vi "IO_csv_writer.vi"(0 "info_sheet":string, 1 "path":path, 2 "y_data_arr":dbl[][](array[numeric]), 3 "x_data_arr":dbl[][](array[numeric])) -> ()   [LabVIEW 2014]
uses:
  dll/csv_operator.dll
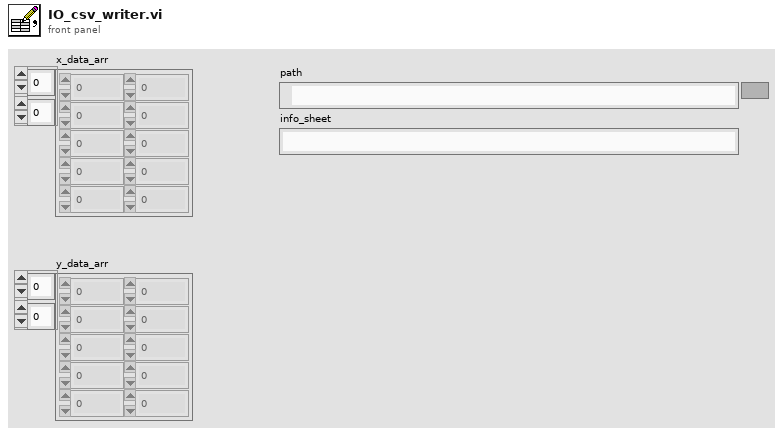
[diagram p1: front panel]
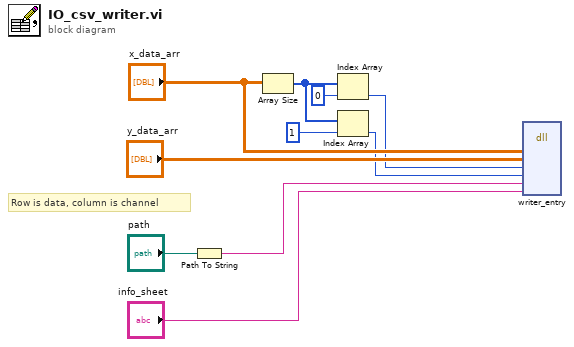
[diagram p0: block diagram]
diagram:
  # "Row is data, column is channel"
  n1 = Path To String(path="path") -> (string=w1:string)
  n2 = Array Size(array="x_data_arr") -> (size(s)=w5:i32[])
  n3 = Index Array(array=w5, index=0) -> (element=w4:i32)
  n4 = Index Array(array=w5, index=1) -> (element=w3:i32)
  n5 = dll-call lib="C:/Users/DrippySummer/Documents/LabVIEW Data/SavaData/keithley_general_client/dll/csv_operator.dll" fn="writer_entry"("x_data_array"="x_data_arr", "y_data_array"="y_data_arr", "row_num"=w4, "col_num"=w3, "path"=w1, "info_sheet"="info_sheet") -> ()  [unwired: 10 in, 2 out]
